vi "Generate ATS Excel Report.vi"(0 "Test Info":string[][](table), 1 "Test_End_Time":string="70", 2 "ATS Number":string="70", 3 "Test_Start_Time":string="20", 5 "Test Table":string[][](table)=[[""]], 7 "Cal Date":string="70", 9 "template":path=path "C:/Users/TMTEST/Desktop/builds/Hartwell/Torque Motor Tester/Template.xlsx", 11 "error in (no error)":errorcluster) -> (15 "error out":errorcluster)   [LabVIEW 2018]
doc: "This example shows how to generate a report from a template. The template contains a preformatted table and a preformatted graph which are updated with Append Table to Report.vi and Excel Update Graph.vi."
uses:
  Controls/Test Table Organization.ctl
  <vilib>/Utility/NIReport.llb/Report Type.ctl
  <vilib>/addons/_office/excel.llb/Excel Easy Table (str).vi
  <vilib>/Utility/NIReport.llb/NI_report.lvclass
  <vilib>/addons/_office/NI_ReportGenerationToolkit.lvlib
  <vilib>/Utility/NIReport.llb/Excel/NI_Excel.lvclass
  <vilib>/Utility/NIReport.llb/NI_ReportGenerationCore.lvlib
panel:
  in  "Test Data Row Documentation":T1
  # "This example shows how to generate a report from a template using either the Excel Report Generation VIs or the MS Office Report Express VI. The template contains several named cells which are used to place data in the appropriate positions in the template."
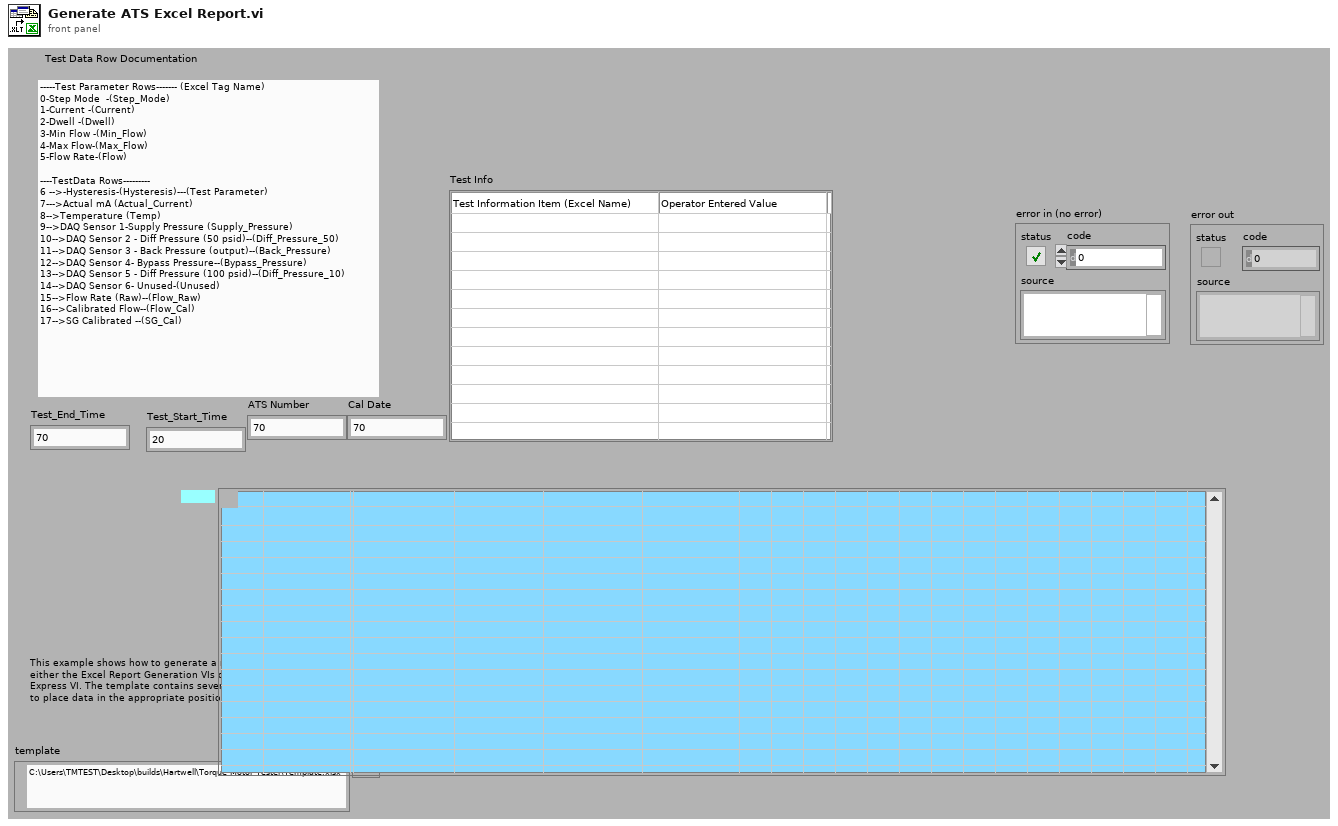
[diagram p1: front panel]
types:
  T1 = typedef "Test Table Organization.ctl" = string
  T2 = typedef "NI_ReportGenerationCore.lvlib/Report Type.ctl" = enum16{"HTML", "Word", "Excel"}
  T3 = enum16{"maximized", "minimized", "normal", "no change"}
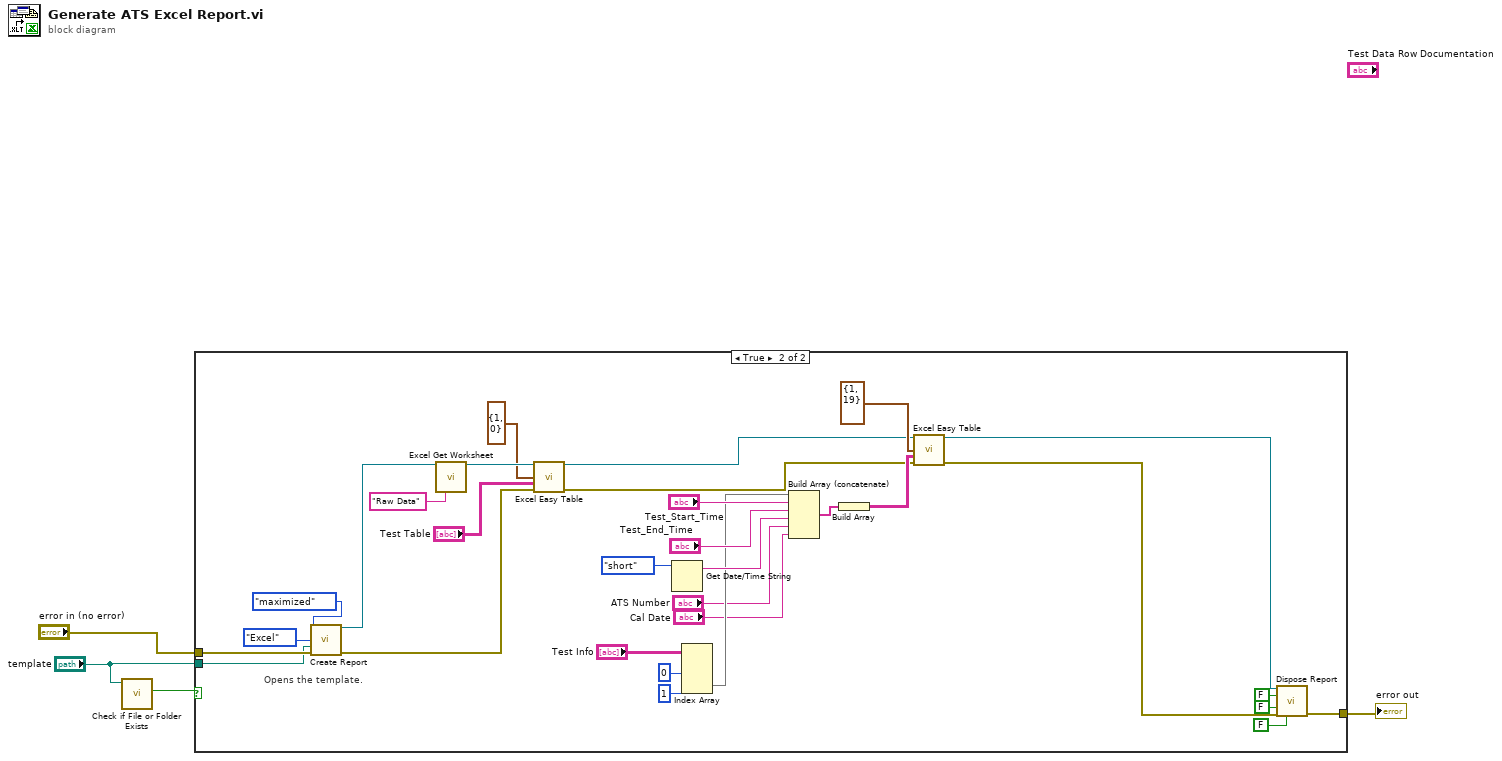
[diagram p0: block diagram]
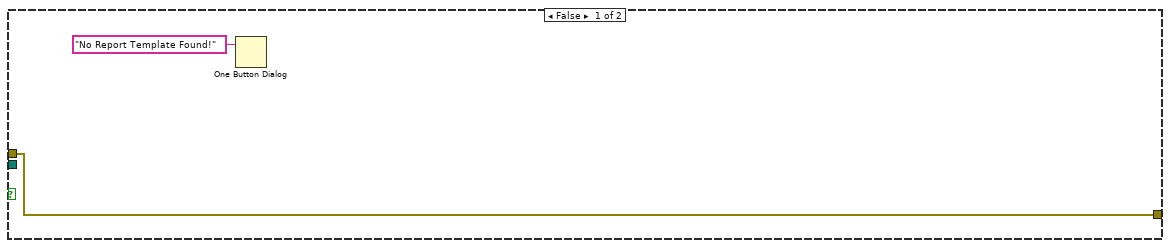
[diagram p2: hidden frame]
diagram:
  n1 = call <vilib>:"Check if File or Folder Exists.vi"("path"="template") -> ("file or folder exists?"=w3:bool)  [unwired: 8 in, 2 out]
  n2 = case shown="True" w3 {
    tunnel: "template" -> [_ w11]
    tunnel: [w5 w13] -> w2
    tunnel: "error in (no error)" -> [w5 w12]
    frame False {
      n3 = One Button Dialog(message="No Report Template Found!") -> ()  [unwired: 1 in, 1 out]
    }
    frame True {
      # "Opens the template."
      n4 = call <vilib>:"Create Report.vi"("window state (normal)"=T3."maximized", "report type"=Report_Type."Excel", "template (empty)"=w11, "error in (no error)"=w12) -> ("report out"=w26:refnum<class "NI_report.lvclass">, "error out"=w10:errorcluster)  [unwired: 10 in]
      n5 = call <vilib>:"Excel Get Worksheet.vi"("report in"=w26, "name (\"\")"="Raw Data" ("name (\"\")")) -> ("report out"=w31:refnum<class "NI_report.lvclass">)  [unwired: 12 in, 1 out]
      n6 = call-poly <vilib>:"Excel Easy Table.vi"("report in"=w31, "start (0, 0)"=cluster{"row":i32, "column":i32} {"row"=1, "column"=0}, "text data"="Test Table", "error in (no error)"=w10) -> ("report out"=w18:refnum<class "NI_report.lvclass">, "error out"=w9:errorcluster)  [unwired: 7 in, 3 out]
      n7 = Get Date/Time String(date format (0)=enum16{"short", "long", "abbreviated"}."short") -> (date string=w23:string)  [unwired: 2 in, 1 out]
      n8 = Index Array(array="Test Info", index (col) #1=0 ("disabled index (col)"), index (col) #2=1 ("index (col)")) -> (element #2=w19:string[])  [unwired: 2 in, 1 out]
      n9 = Build Array (concatenate)(w19, "Test_Start_Time", "Test_End_Time", w23, "ATS Number", "Cal Date") -> (w21:string[])
      n10 = Build Array(w21) -> (w20:string[][])
      n11 = call-poly <vilib>:"Excel Easy Table.vi"("report in"=w18, "start (0, 0)"=cluster{"row":i32, "column":i32} {"row"=1, "column"=19}, "text data"=w20, "error in (no error)"=w9) -> ("report out"=w8:refnum<class "NI_report.lvclass">, "error out"=w7:errorcluster)  [unwired: 7 in, 3 out]
      n12 = call-dynamic "Dispose Report.vi"("report in"=w8, "wait until printing completed? (T)"=FALSE, "save changes? (F)"=FALSE, "error in (no error)"=w7, "close report? (T)"=FALSE ("Close Report? (T)")) -> ("error out"=w13:errorcluster)  [unwired: 10 in]
    }
  }
  "error out" <- w2
